vi "cDAQ_VI_Leo.vi"() -> ()   [LabVIEW 2022 SP3]
uses:
  <vilib>/Analysis/baseanly.llb/Mean (DBL).vi
  STOP_GLOBAL.vi
  <vilib>/Analysis/NI_AALBase.lvlib
panel:
  in  "number of samples":i32=60
  in  "rate":dbl=60.0
  out "Temperature":dbl[](graph)
  out "Temperature":dynamicdata(graph)
  out "Thrust":dbl[](graph)
  out "Numeric 2":i32
  out "Numeric":i32
  out "Thrust lb":dynamicdata(graph)
  in  "Types of Testing":enum32{"Test Firing", "Cold Flow Rig"}(tab)
  out "Saving Data":bool
  out "Filename Out 4":path caption="Filename Out"
  in  "Enable":bool=TRUE
  in  "Filename 4":path=path "C:/1. Rocket Research Project/CollectedData/Calibrations/Thrust_Testing_7.lvm" caption="Filename"
  out "Saving Data":bool
  out "Filename Out 3":path caption="Filename Out"
  in  "Enable":bool=TRUE
  in  "Collect Data?":bool=TRUE caption="Enable"
  out "Filename Out":path
  out "Saving Data":bool
  in  "Filename":path=path "C:/1. Rocket Research Project/CollectedData/Calibrations/Thrust_Testing_7.lvm"
  in  "Filename 3":path=path "C:/1. Rocket Research Project/CollectedData/Calibrations/Thrust_Testing_7.lvm" caption="Filename"
  in  "Enable":bool=TRUE
  out "Filename Out 2":path caption="Filename Out"
  in  "Filename 2":path=path "C:/1. Rocket Research Project/CollectedData/Calibrations/Thrust_Testing_7.lvm" caption="Filename"
  in  "Collect Data? 2":bool=TRUE caption="Enable"
  out "Saving Data 2":bool caption="Saving Data"
  out "Saving Data":bool
  out "Filename Out 5":path caption="Filename Out"
  in  "Filename 5":path=path "C:/1. Rocket Research Project/CollectedData/Calibrations/Thrust_Testing_7.lvm" caption="Filename"
  in  "Rate 9237":dbl=25000.0
  in  "Samples 9237":i32=25000
  in  "Rate 9219":dbl=60.0
  in  "Samples 9219":i32=60
  out "Supply Pressure PSI":dynamicdata(graph)
  out "4th Channel NI 9219":dynamicdata(graph)
  out "Mass Flow":dbl[](graph)
  out "Mass Flow L/min":dynamicdata(graph)
  out "Chamber Pressure":dbl[](graph)
  out "Supply Pressure":dbl[](graph)
  out "Chamber Pressure PSI":dynamicdata(graph)
  # "DATA LOGGING INFORMATION"
  # "ANALOG VOLTAGE OUTPUT"
  # "RESULTS"
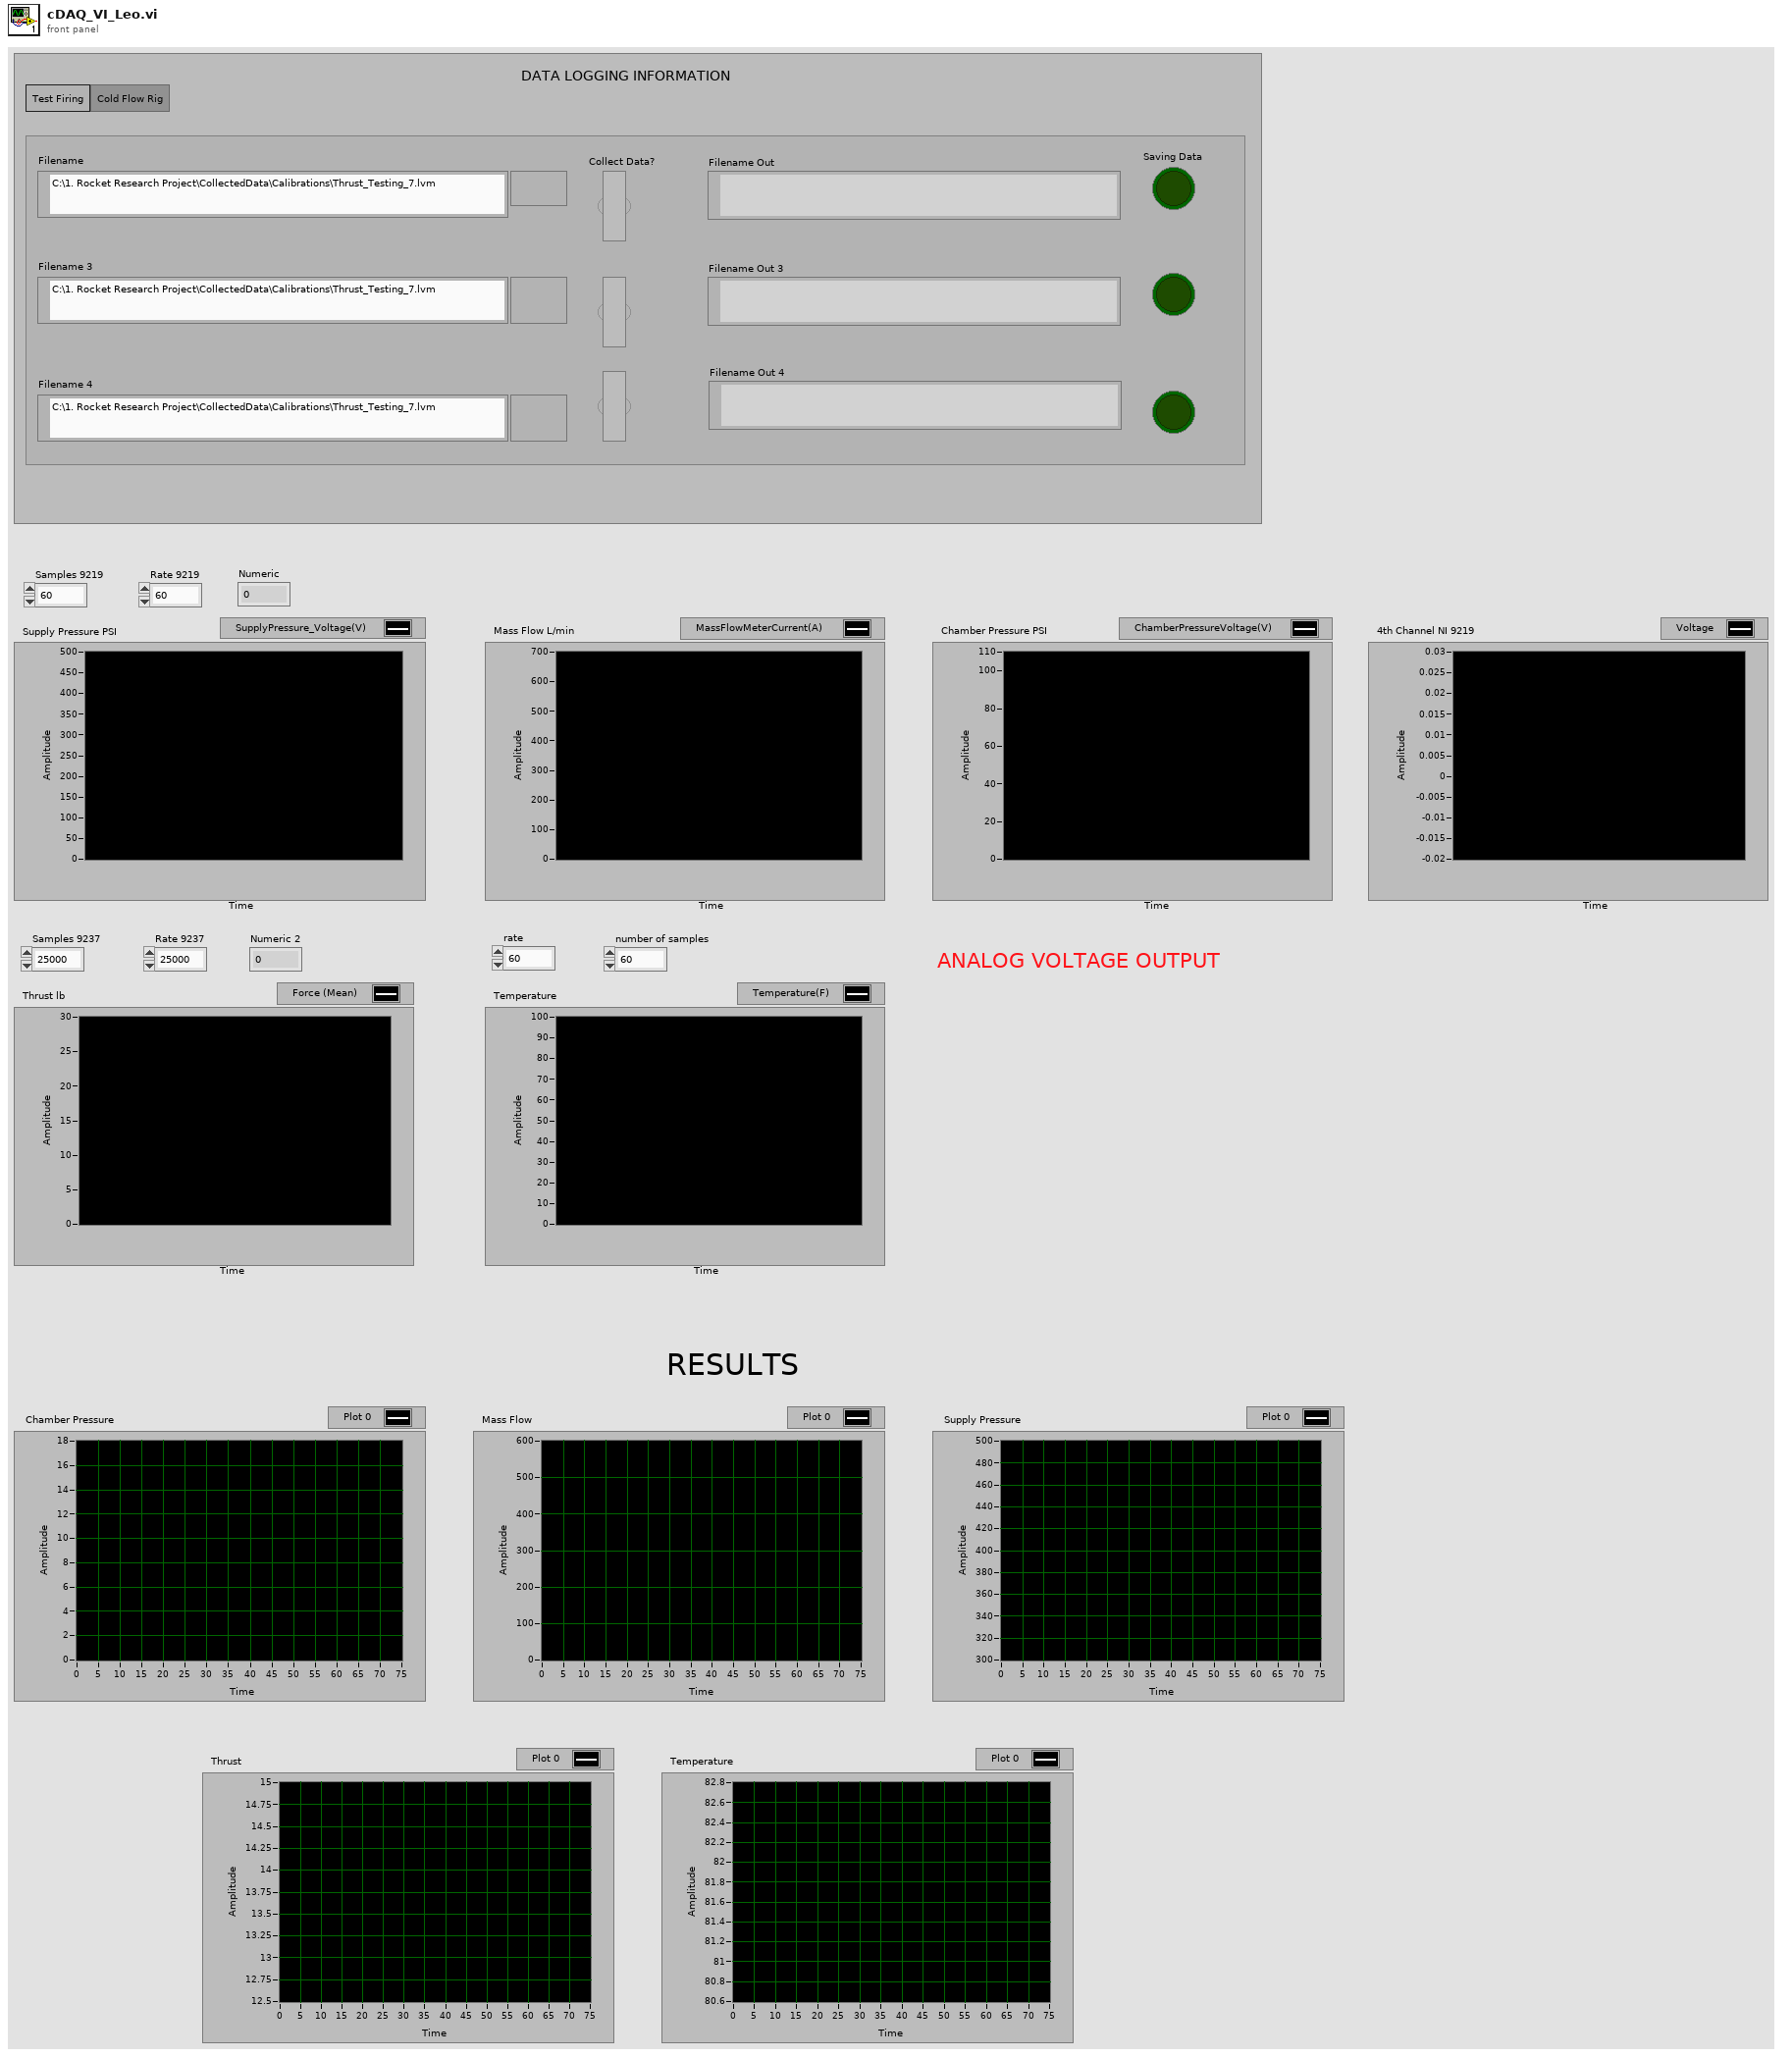
[diagram p1: front panel]
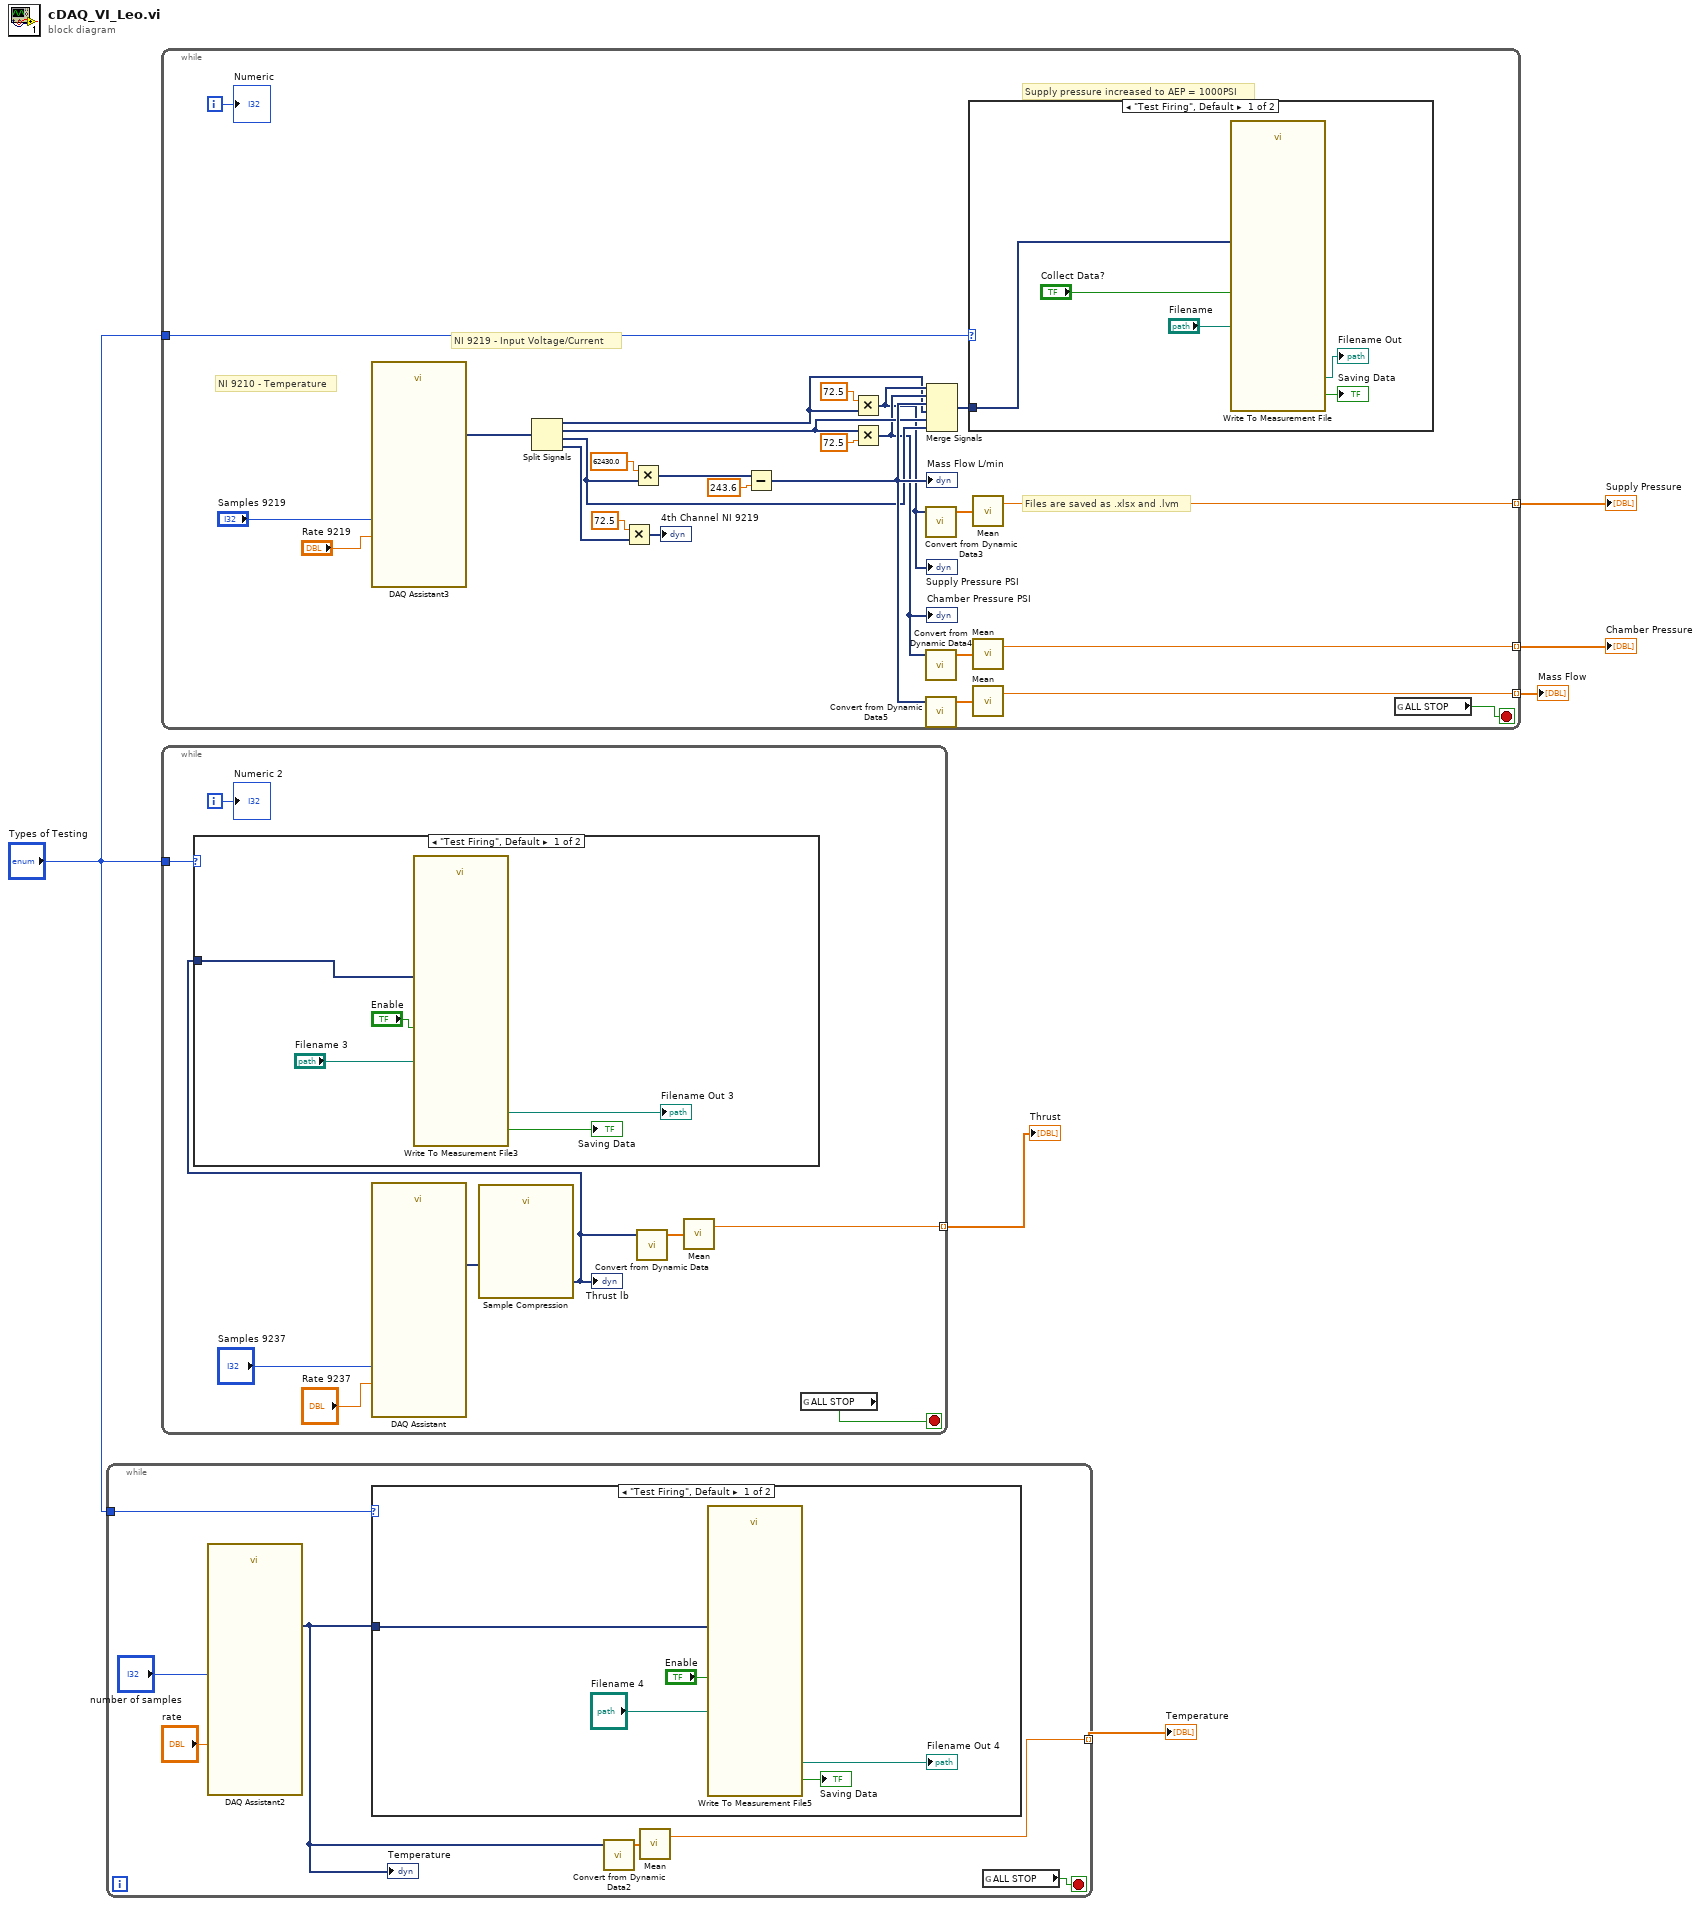
[diagram p0: block diagram]
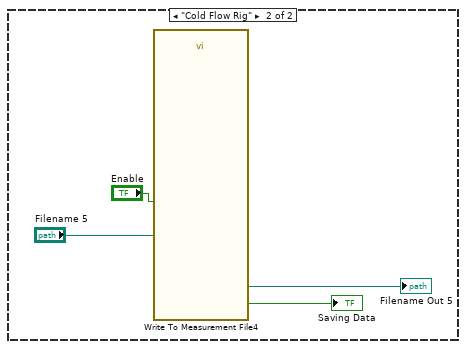
[diagram p3: hidden frame]
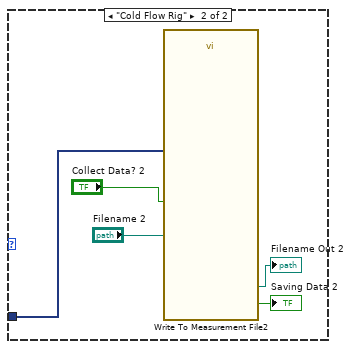
[diagram p4: hidden frame]
diagram:
  n1 = while {
    tunnel: "Types of Testing" -> [w12]
    tunnel: [w10] -> w1 mode=indexing
    stop <- w13 stop-if-true
    n2 = call "DAQ Assistant2"("rate"="rate", "number of samples"="number of samples") -> ("data"=w7:dynamicdata)  [unwired: 14 in, 3 out]
    "Temperature" <- w7
    n3 = case shown="\"Test Firing\", Default" w12 {
      tunnel: w7 -> [w14 _]
      frame "Test Firing", Default {
        n4 = call "Write To Measurement File5"("Signals"=w14, "Enable"="Enable", "Filename"="Filename 4") -> ("Filename Out"=→"Filename Out 4":path, "Saving Data"=→"Saving Data":bool)  [unwired: 14 in, 1 out]
      }
      frame "Cold Flow Rig" {
      }
    }
    n5 = call "Convert from Dynamic Data2"("Dynamic Data Type"=w7) -> ("Array"=w11:dbl[])  [unwired: 3 in]
    n6 = call-poly <vilib>:"Mean.vi"("X"=w11) -> ("mean"=w10:dbl)  [unwired: 1 out]
    n7 = global read "STOP_GLOBAL.vi" "ALL STOP"() -> (w13:bool)
  }
  "Temperature" <- w1
  n8 = while {
    tunnel: [w44] -> w6 mode=indexing
    tunnel: [w19] -> w5 mode=indexing
    tunnel: [w35] -> w4 mode=indexing
    tunnel: "Types of Testing" -> [w22]
    i -> [w20]
    stop <- w31 stop-if-true
    # "Files are saved as .xlsx and .lvm"
    # "NI 9210 - Temperature"
    # "Supply pressure increased to AEP = 1000PSI"
    # "NI 9219 - Input Voltage/Current"
    n9 = call "DAQ Assistant3"("rate"="Rate 9219", "number of samples"="Samples 9219") -> ("data"=w37:dynamicdata)  [unwired: 14 in, 3 out]
    n10 = Split Signals(w37) -> (w28:dynamicdata, w33:dynamicdata, w32:dynamicdata, w27:dynamicdata)  [unwired: 4 in]
    n11 = Multiply(x=72.5, y=w27) -> (x*y=→"4th Channel NI 9219":dynamicdata)
    n12 = Multiply(x=62430.0, y=w32) -> (x*y=w38:dynamicdata)
    n13 = Subtract(x=w38, y=243.6) -> (x-y=w34:dynamicdata)
    "Mass Flow L/min" <- w34
    n14 = Multiply(x=72.5, y=w28) -> (x*y=w29:dynamicdata)
    "Supply Pressure PSI" <- w29
    n15 = Multiply(x=w33, y=72.5 ("x")) -> (x*y=w30:dynamicdata)
    "Chamber Pressure PSI" <- w30
    n16 = call "Convert from Dynamic Data3"("Dynamic Data Type"=w29) -> ("Array"=w36:dbl[])  [unwired: 3 in]
    n17 = call "Convert from Dynamic Data4"("Dynamic Data Type"=w30) -> ("Array"=w45:dbl[])  [unwired: 3 in]
    n18 = call "Convert from Dynamic Data5"("Dynamic Data Type"=w34) -> ("Array"=w41:dbl[])  [unwired: 3 in]
    n19 = Merge Signals(w29, w30, w34, w28, w33, w32) -> (w21:dynamicdata)
    n20 = case shown="\"Test Firing\", Default" w22 {
      tunnel: w21 -> [w46 w51]
      frame "Test Firing", Default {
        n21 = call "Write To Measurement File"("Signals"=w46, "Enable"="Collect Data?", "Filename"="Filename") -> ("Filename Out"=→"Filename Out":path, "Saving Data"=→"Saving Data":bool)  [unwired: 14 in, 1 out]
      }
      frame "Cold Flow Rig" {
        n22 = call "Write To Measurement File2"("Signals"=w51, "Enable"="Collect Data? 2", "Filename"="Filename 2") -> ("Filename Out"=→"Filename Out 2":path, "Saving Data"=→"Saving Data 2":bool)  [unwired: 14 in, 1 out]
      }
    }
    n23 = call-poly <vilib>:"Mean.vi"("X"=w36) -> ("mean"=w35:dbl)  [unwired: 1 out]
    n24 = call-poly <vilib>:"Mean.vi"("X"=w45) -> ("mean"=w44:dbl)  [unwired: 1 out]
    n25 = call-poly <vilib>:"Mean.vi"("X"=w41) -> ("mean"=w19:dbl)  [unwired: 1 out]
    n26 = global read "STOP_GLOBAL.vi" "ALL STOP"() -> (w31:bool)
    "Numeric" <- w20
  }
  "Supply Pressure" <- w4
  "Chamber Pressure" <- w6
  "Mass Flow" <- w5
  n27 = while {
    tunnel: "Types of Testing" -> [w59]
    tunnel: [w57] -> w2 mode=indexing
    i -> [w60]
    stop <- w64 stop-if-true
    n28 = call "DAQ Assistant"("rate"="Rate 9237", "number of samples"="Samples 9237") -> ("data"=w61:dynamicdata)  [unwired: 14 in, 3 out]
    n29 = call "Sample Compression"("Signals"=w61) -> ("Mean"=w56:dynamicdata)  [unwired: 8 in, 2 out]
    "Thrust lb" <- w56
    n30 = case shown="\"Test Firing\", Default" w59 {
      tunnel: w56 -> [w65 _]
      frame "Test Firing", Default {
        n31 = call "Write To Measurement File3"("Signals"=w65, "Enable"="Enable", "Filename"="Filename 3") -> ("Filename Out"=→"Filename Out 3":path, "Saving Data"=→"Saving Data":bool)  [unwired: 14 in, 1 out]
      }
      frame "Cold Flow Rig" {
        n32 = call "Write To Measurement File4"("Enable"="Enable", "Filename"="Filename 5") -> ("Filename Out"=→"Filename Out 5":path, "Saving Data"=→"Saving Data":bool)  [unwired: 15 in, 1 out]
      }
    }
    n33 = call "Convert from Dynamic Data"("Dynamic Data Type"=w56) -> ("Array"=w58:dbl[])  [unwired: 3 in]
    n34 = call-poly <vilib>:"Mean.vi"("X"=w58) -> ("mean"=w57:dbl)  [unwired: 1 out]
    n35 = global read "STOP_GLOBAL.vi" "ALL STOP"() -> (w64:bool)
    "Numeric 2" <- w60
  }
  "Thrust" <- w2
